vi "NI6071E.Connect.vi"(0 "i ref in":refnum<vi>, 1 "Node name":string, 2 "Port":i32=6341, 4 "timeout ms (60000)":i32=60000, 5 "error in (no error)":errorcluster) -> (14 "i ref out":refnum<vi>, 19 "error out":errorcluster)   [LabVIEW 2014, in "NI6071E.lvlib"]
uses:
  NI6071E.lvlib
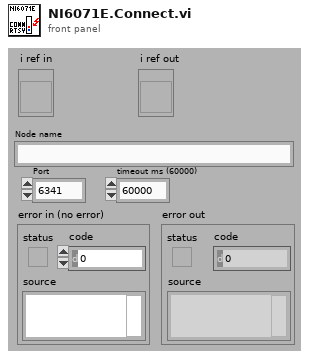
[diagram p1: front panel]
types:
  T1 = typedef "NI6071E.lvlib/NI6071E.i attribute.ctl" = cluster{"NI6071E Server":string, "Port":u16, "NI6071E Config":T2, "NI6071E Start":T3, "Waveforms":waveform(dbl)[], "RT Error":errorcluster, "NI6071E Read":T4, "connection ID":refnum<k5>, "DAQ Status":string, "device (1)":i16, "DAQ Status Service ID":i32}
  T2 = typedef "NI6071E.lvlib/NI6071EConfig.ctl" = cluster{"device (1)":i16, "channels (0)":tag[], "buffer size (1000 scans)":i32, "[number of buffers] (1)":i32, "measurement mode structure":cluster{"measurement mode":u16, "reserved":u32}, "input limits (no change)":cluster{"high limit (0.0)":sgl, "low limit (0.0)":sgl}[], "coupling & input config (no change:0)":cluster{"coupling (no change:0)":enum16{"no change", "DC", "AC", "GND", "internal ref."}, "input config (no change:0)":u16}[]}
  T3 = typedef "NI6071E.lvlib/NI6071EStart.ctl" = cluster{"scan rate (40000 scans/sec)":sgl, "trigger type (analog)":enum16{"no trigger", "analog", "digital A", "digital A & B", "scan clock gate"}, "edge or slope \n(rising)":enum16{"no change", "rising", "falling"}, "number of buffers to acquire (1)":i32, "analog chan (PFI0) & level (2.00)":cluster{"trigger channel (empty)":string, "level (0.0)":sgl}, "[additional trig params]":cluster{"hysteresis (0.0)":sgl, "coupling (no change:0)":enum16{"no change", "DC", "AC"}, "delay (0 sec)":sgl, "skip count (0)":i32, "time limit (0 sec)":sgl}}
  T4 = typedef "NI6071E.lvlib/NI6071ERead.ctl" = cluster{"time limit in sec (-1:auto calculate)":sgl, "number of scans to read (-1:all)":i32}
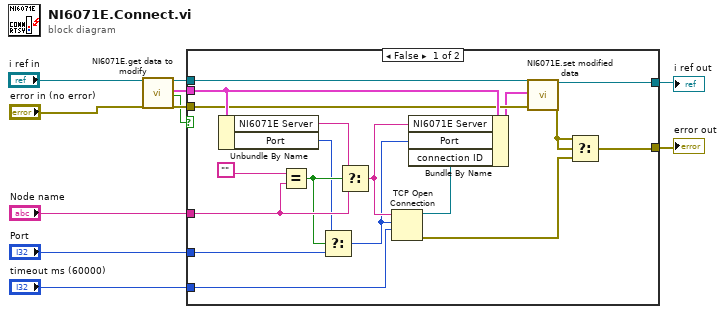
[diagram p0: block diagram]
diagram:
  n1 = call "NI6071E.get data to modify.vi"("i ref in"="i ref in", "error in (no error)"="error in (no error)") -> ("i ref out"=w5:refnum<vi>, "i attribute"=w8:T1, "timed out"=w1:bool, "error out"=w6:errorcluster)  [unwired: 14 in]
  n2 = case shown="False" w1 {
    tunnel: "Node name" -> [w28 _]
    tunnel: w8 -> [w26 _]
    tunnel: "Port" -> [w22 _]
    tunnel: w6 -> [w19 w30]
    tunnel: w5 -> [w18 w31]
    tunnel: [w17 w31] -> w4
    tunnel: [w14 w30] -> w3
    tunnel: "timeout ms (60000)" -> [w12 _]
    frame False {
      n3 = Unbundle By Name(w26) -> ("NI6071E Server"=w27:string, "Port"=w23:u16)
      n4 = Equal?(x="", y=w28) -> (x = y?=w24:bool)
      n5 = Select(t=w23, s=w24, f=w22) -> (s? t:f=w21:i32)
      n6 = Select(t=w27, s=w24, f=w28) -> (s? t:f=w25:string)
      n7 = TCP Open Connection(address=w25, remote port or service name=w21, timeout ms (60000)=w12) -> (connection ID=w20:refnum<k5>, error out=w15:errorcluster)  [unwired: 2 in]
      n8 = Bundle By Name(cluster=w26, "NI6071E Server"=w25, "Port"=w21, "connection ID"=w20) -> (w13:T1)
      n9 = call "NI6071E.set modified data.vi"("i ref in"=w18, "i attribute"=w13, "error in (no error)"=w19) -> ("i ref out"=w17:refnum<vi>, "error out"=w16:errorcluster)  [unwired: 15 in]
      n10 = Select(t=w16, s=w16, f=w15) -> (s? t:f=w14:errorcluster)
    }
    frame True {
    }
  }
  "i ref out" <- w4
  "error out" <- w3
